vi "Agilent 6000 Series Acquire Continuous Waveform.vi"() -> ()   [LabVIEW 2017]
doc: "This example shows how to acquire a waveform continuously on a single channel."
uses:
  <instrlib>/Agilent 6000 Series/Public/Data/Read Single Waveform.vi
  <instrlib>/Agilent 6000 Series/Agilent 6000 Series.lvlib
panel:
  in  "Source (0: Channel 1)":u16(ring) items=["Channel 1", "Channel 2", "Channel 3", "Channel 4"]
  in  "stop":bool
  in  "Probe Attenuation (1.0)":dbl=1.0
  in  "Timeout (10000 ms)":u32=10000
  out "Waveform Data":waveform(dbl)(graph)
  in  "VISA resource name":refnum<visa-resource-name>
  # "(c) 2009-2015 National Instruments.  ALL RIGHTS RESERVED."
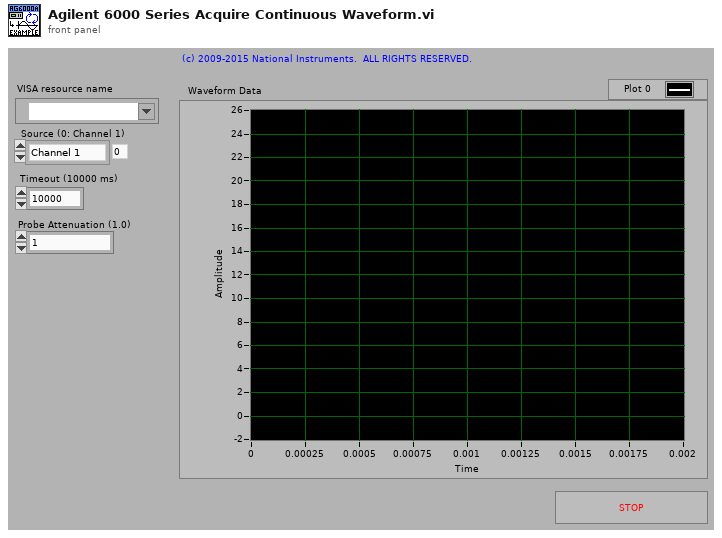
[diagram p1: front panel]
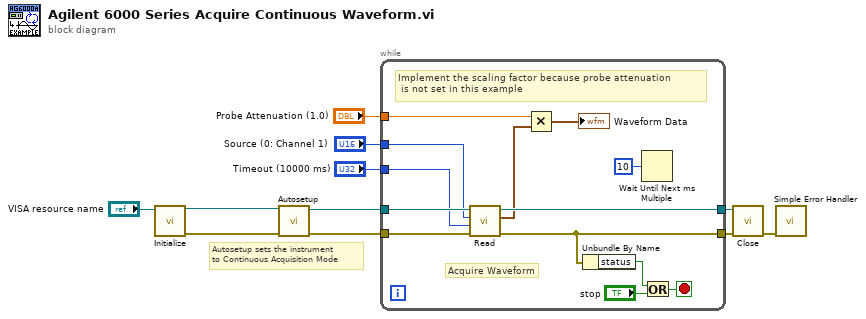
[diagram p0: block diagram]
diagram:
  # "Autosetup sets the instrument\nto Continuous Acquisition Mode"
  n1 = call <instrlib>:"Initialize.vi"("VISA resource name"="VISA resource name") -> ("error out"=w6:errorcluster, "VISA resource name out"=w5:refnum<visa-resource-name>)  [unwired: 9 in]
  n2 = call <instrlib>:"Autosetup.vi"("error in (no error)"=w6, "VISA resource name"=w5) -> ("error out"=w2:errorcluster, "VISA resource name out"=w3:refnum<visa-resource-name>)  [unwired: 8 in]
  n3 = while {
    tunnel: w3 -> [w24]
    tunnel: w2 -> [w23]
    tunnel: [w22] -> w10
    tunnel: [w16] -> w9
    tunnel: "Timeout (10000 ms)" -> [w21]
    tunnel: "Probe Attenuation (1.0)" -> [w20]
    tunnel: "Source (0: Channel 1)" -> [w12]
    stop <- w17 stop-if-true
    # "Implement the scaling factor because probe attenuation\n is not set in this example"
    # "Acquire Waveform"
    n4 = call-poly <instrlib>:"Read.vi"("error in (no error)"=w23, "Timeout (10000 ms)"=w21, "Source (0: Channel 1)"=w12, "VISA resource name"=w24) -> ("error out"=w16:errorcluster, "Waveform Data"=w13:waveform(dbl), "VISA resource name out"=w22:refnum<visa-resource-name>)  [unwired: 5 in]
    n5 = Multiply(x=w20, y=w13) -> (x*y=→"Waveform Data":waveform(dbl))
    n6 = Unbundle By Name(w16) -> ("status"=w15:bool)
    n7 = Wait Until Next ms Multiple(millisecond multiple=u32 10) -> ()  [unwired: 1 out]
    n8 = Or(x=w15, y="stop") -> (x .or. y?=w17:bool)
  }
  n9 = call <instrlib>:"Close.vi"("error in (no error)"=w9, "VISA resource name"=w10) -> ("error out"=w11:errorcluster)  [unwired: 9 in]
  n10 = call <vilib>:"Simple Error Handler.vi"("error in (no error)"=w11) -> ()  [unwired: 4 in, 5 out]
